vi "Initialize.vi"(8 "error in":errorcluster, 11 "Plugin in":refnum<class "MP710995.lvclass">) -> (0 "error out":errorcluster, 3 "Plugin out":refnum<class "MP710995.lvclass">)   [LabVIEW 2025, in "MP710995.lvlib" / "MP710995.lvclass"]
uses:
  MP710995.lvclass
  C:/Program Files/National Instruments/LabVIEW 2025/vi.lib/FlexLogger/SDK/PluginSDK.lvlibp/PEFClasses/SDK/Plugin/Plugin.lvclass
  <vilib>/FlexLogger/SDK/PluginSDK.lvlibp/PEFClasses/SDK/Processing Element/Timing Parameters.ctl
  <vilib>/FlexLogger/SDK/PluginSDK.lvlibp/PEFClasses/SDK/Processing Element/Timing Method.ctl
  <vilib>/FlexLogger/SDK/PluginSDK.lvlibp/PEFClasses/SDK/Channel/Data Type.ctl
  MP710995.lvclass/MP710995.ctl
  <vilib>/FlexLogger/SDK/PluginSDK.lvlibp/PEFClasses/SDK/Setpoint Consumer Channel/Setpoint Consumer Channel.lvclass
  C:/Program Files/National Instruments/LabVIEW 2025/vi.lib/FlexLogger/SDK/PluginSDK.lvlibp/PEFClasses/SDK/Channel/Channel.lvclass
  <vilib>/FlexLogger/SDK/PluginSDK.lvlibp/PEFClasses/SDK/Producer Channel/Producer Channel.lvclass
  <vilib>/FlexLogger/SDK/PluginSDK.lvlibp/PEFClasses/SDK/Plugin/ParameterAccess/Write String.vi
  <vilib>/FlexLogger/SDK/PluginSDK.lvlibp/PEFClasses/SDK/Setpoint Consumer Channel/Create Setpoint Consumer Channel.vi
  <vilib>/FlexLogger/SDK/PluginSDK.lvlibp/PEFClasses/SDK/Producer Channel/Create Producer Channel_v2.vi
  <vilib>/FlexLogger/SDK/PluginSDK.lvlibp/PEFClasses/SDK/Plugin/Plugin.lvclass
  <vilib>/FlexLogger/SDK/PluginSDK.lvlibp/PEFClasses/SDK/Channel/Channel.lvclass
  <vilib>/FlexLogger/SDK/PluginSDK.lvlibp/PEFClasses/SDK/Processing Element/Processing Element.lvclass
  <vilib>/FlexLogger/SDK/PluginSDK.lvlibp
  <vilib>/FlexLogger/SDK/PluginSDK.lvlibp/PEFClasses/SDK/Channel/ParameterAccess/Write DBL.vi
  <vilib>/FlexLogger/SDK/PluginSDK.lvlibp/PEFClasses/SDK/Channel/ParameterAccess/Write Boolean.vi
  Device Info.ctl
  C:/Program Files/National Instruments/LabVIEW 2025/vi.lib/FlexLogger/SDK/PluginSDK.lvlibp/PEFClasses/SDK/Consumer Channel/Consumer Channel.lvclass
  C:/Program Files/National Instruments/LabVIEW 2025/vi.lib/FlexLogger/SDK/PluginSDK.lvlibp/PEFClasses/SDK/Setpoint Consumer Channel/Setpoint Consumer Channel.lvclass
  C:/Program Files/National Instruments/LabVIEW 2025/vi.lib/FlexLogger/SDK/PluginSDK.lvlibp/PEFClasses/SDK/Processing Element/Processing Element.lvclass
  C:/Users/Steve/Documents/Git/MP710995-Plugin/Source/MP710995/MP710995.lvclass
panel:
  # "C:\\Program Files\\National Instruments\\LabVIEW 2025\\resource\\FlexLogger\\SDK\\PluginEnvironmentSimulator"
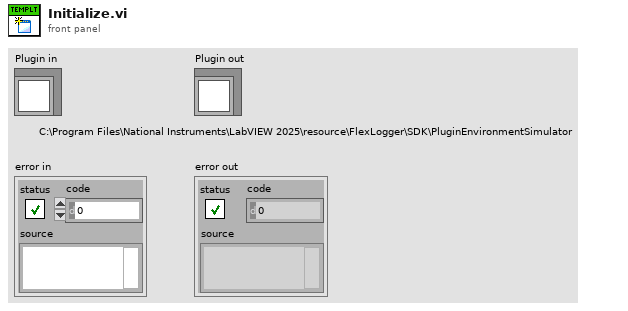
[diagram p1: front panel]
types:
  T1 = cluster{"Output":bool, "Current Limit":dbl, "Voltage":dbl, "Measured Voltage":dbl, "Measured Current":dbl, "OCP":bool}[]
  T2 = typedef "PluginSDK.lvlibp/Channel.lvclass/Data Type.ctl" = enum16{"Wfm (DBL)", "Wfm (Digital)"}
  T3 = typedef "PluginSDK.lvlibp/Processing Element.lvclass/Timing Parameters.ctl" = cluster{"Timing Method":T4, "Timing Period (ms)":i32}
  T4 = typedef "PluginSDK.lvlibp/Processing Element.lvclass/Timing Method.ctl" = enum16{"Periodic", "Immediate", "On Data Ready", "Triggered"}
  T5 = typedef "Device Info.ctl" = cluster{"Device Name":string, "Serial Number":string, "Channels":cluster{"Output":bool, "Current Limit":dbl, "Voltage":dbl, "OVP":bool, "OCP":bool}[]}
  T6 = cluster{"Output":bool, "Current Limit":dbl, "Voltage":dbl, "OVP":bool, "OCP":bool}[]
  T7 = cluster{"Output":bool, "Current Limit":dbl, "Voltage":dbl, "OVP":bool, "OCP":bool}
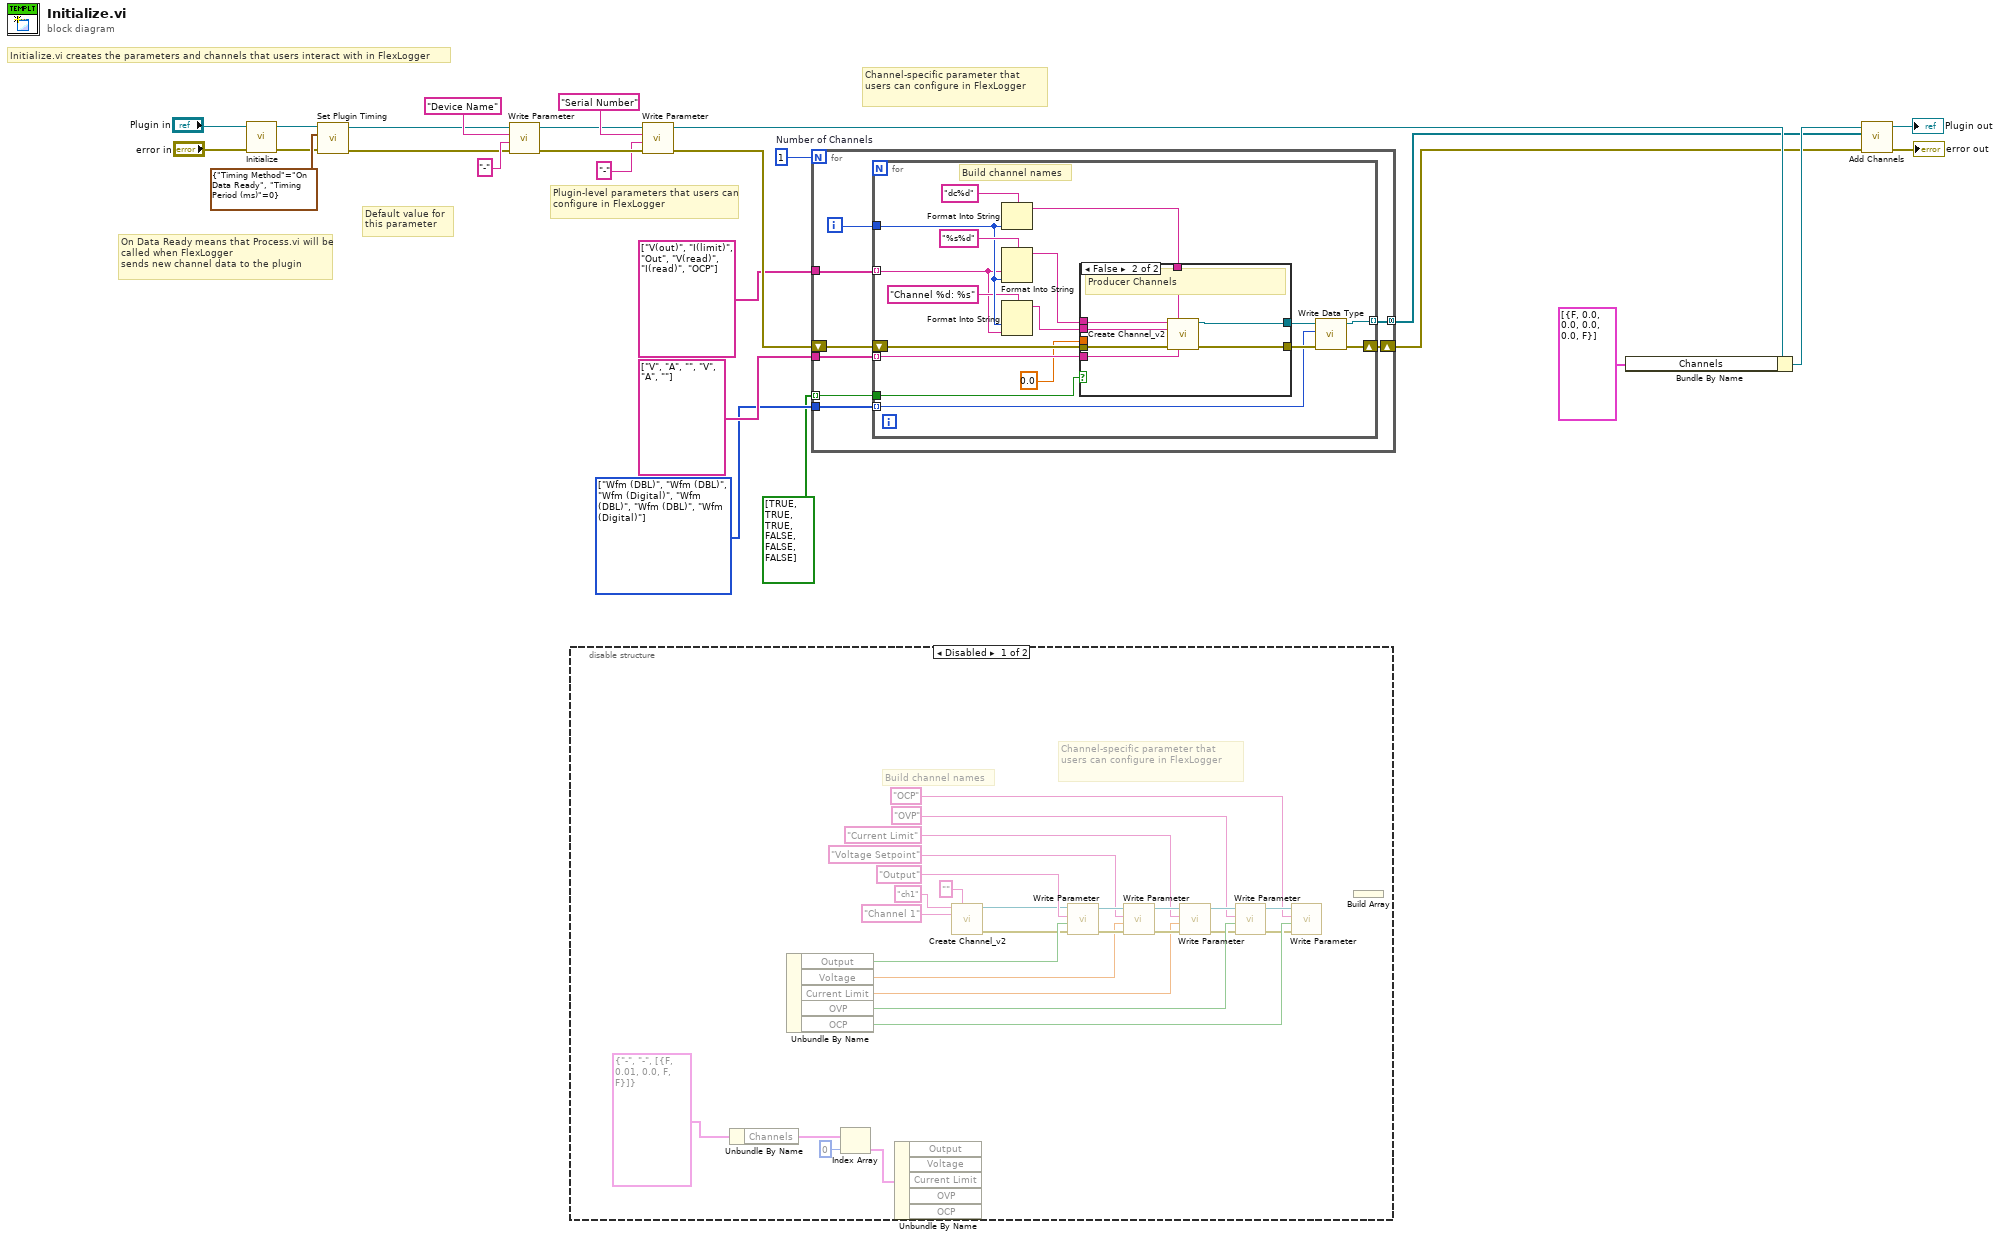
[diagram p0: block diagram]
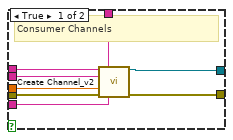
[diagram p2: hidden frame]
diagram:
  w5 = T2[] [enum."Wfm (DBL)", enum."Wfm (DBL)", enum."Wfm (Digital)", enum."Wfm (DBL)", enum."Wfm (DBL)", enum."Wfm (Digital)"] items=["Wfm (DBL)", "Wfm (Digital)"]
  w8 = 1  # Number of Channels
  # "Channel-specific parameter that users can configure in FlexLogger"
  # "Default value for this parameter"
  # "Plugin-level parameters that users can configure in FlexLogger"
  # "On Data Ready means that Process.vi will be called when FlexLogger \nsends new channel data to the plugin"
  # "Initialize.vi creates the parameters and channels that users interact with in FlexLogger"
  n1 = call-parent "Initialize.vi"("error in (no error)"="error in", "Plugin in"="Plugin in") -> ("error out"=w19:errorcluster, "Plugin out"=w18:refnum<class "MP710995.lvclass">)  [unwired: 8 in]
  n2 = call <vilib>:"Set Plugin Timing.vi"("error in (no error)"=w19, "Timing Parameters"=T3 {"Timing Method"=enum."On Data Ready", "Timing Period (ms)"=0}, "Plugin in"=w18) -> ("error out"=w11:errorcluster, "Plugin out"=w12:refnum<class "MP710995.lvclass">)  [unwired: 7 in]
  n3 = call-poly <vilib>:"Write Parameter.vi"("error in (no error)"=w11, "Value"="-", "Name"="Device Name", "Plugin in"=w12) -> ("error out"=w15:errorcluster, "Plugin out"=w16:refnum<class "MP710995.lvclass">)  [unwired: 6 in]
  n4 = disable-structure shown="Disabled" {
    frame Disabled {
      # "Channel-specific parameter that users can configure in FlexLogger"
      # "Build channel names"
      n5 = Unbundle By Name(T5 {"Device Name"="-", "Serial Number"="-", "Channels"=[{"Output"=FALSE, "Current Limit"=0.01, "Voltage"=0.0, "OVP"=FALSE, "OCP"=FALSE}]}) -> ("Channels"=w30:T6)
      n6 = Unbundle By Name() -> ("Output"=w43:bool, "Voltage"=w49:dbl, "Current Limit"=w47:dbl, "OVP"=w44:bool, "OCP"=w45:bool)  [unwired: 1 in]
      n7 = Index Array(array=w30, index=0) -> (element=w29:T7)
      n8 = Unbundle By Name(w29) -> ()  [unwired: 5 out]
      n9 = call-poly <vilib>:"Create Channel_v2.vi"("Unique Channel Identifier"="ch1" ("format string"), "Display Group"="", "Default Channel Name"="Channel 1" ("format string")) -> ("Setpoint Consumer Channel"=w35:refnum<class "Setpoint Consumer Channel.lvclass">, "error in (no error)"=w33:errorcluster, "error out"=w34:errorcluster)  [unwired: 10 in]
      n10 = call-poly <vilib>:"Write Parameter.vi"("error in (no error)"=w34, "Value"=w43, "Name"="Output", "Channel in"=w35) -> ("error out"=w50:errorcluster, "Channel out"=w51:refnum<class "Setpoint Consumer Channel.lvclass">)  [unwired: 6 in]
      n11 = call-poly <vilib>:"Write Parameter.vi"("error in (no error)"=w50, "Value"=w49, "Name"="Voltage Setpoint", "Channel in"=w51) -> ("error out"=w53:errorcluster, "Channel out"=w52:refnum<class "Setpoint Consumer Channel.lvclass">)  [unwired: 6 in]
      n12 = call-poly <vilib>:"Write Parameter.vi"("error in (no error)"=w53, "Value"=w47, "Name"="Current Limit", "Channel in"=w52) -> ("error out"=w39:errorcluster, "Channel out"=w38:refnum<class "Setpoint Consumer Channel.lvclass">)  [unwired: 6 in]
      n13 = call-poly <vilib>:"Write Parameter.vi"("error in (no error)"=w39, "Value"=w44, "Name"="OVP", "Channel in"=w38) -> ("error out"=w41:errorcluster, "Channel out"=w40:refnum<class "Setpoint Consumer Channel.lvclass">)  [unwired: 6 in]
      n14 = call-poly <vilib>:"Write Parameter.vi"("error in (no error)"=w41, "Value"=w45, "Name"="OCP", "Channel in"=w40) -> ()  [unwired: 6 in, 2 out]
      n15 = Build Array() -> ()  [unwired: 1 in, 1 out]
    }
    frame Enabled {
    }
  }
  n16 = call-poly <vilib>:"Write Parameter.vi"("error in (no error)"=w15, "Value"="-", "Name"="Serial Number", "Plugin in"=w16) -> ("error out"=w13:errorcluster, "Plugin out"=w10:refnum<class "MP710995.lvclass">)  [unwired: 6 in]
  n17 = for {
    N: w8 -> [_]
    tunnel: string[] ["V(out)", "I(limit)", "Out", "V(read)", "I(read)", "OCP"] -> [w60]
    tunnel: string[] ["V", "A", "", "V", "A", ""] -> [w59]
    tunnel: w5 -> [w58]
    shift-right: [w57] -> w3
    shift-left: w13 -> [w62]
    tunnel: [w56] -> w4 mode=concatenating
    tunnel: bool[] [TRUE, TRUE, TRUE, FALSE, FALSE, FALSE] -> [w55] mode=indexing
    i -> [w61]
    n18 = for {
      tunnel: w61 -> [w74]
      tunnel: w60 -> [w72] mode=indexing
      tunnel: w59 -> [w70] mode=indexing
      tunnel: w58 -> [w66] mode=indexing
      shift-right: [w67] -> w57
      shift-left: w62 -> [w79]
      tunnel: [w65] -> w56 mode=indexing
      tunnel: w55 -> [w63]
      # "Build channel names"
      n19 = Format Into String(format string="dc%d", w74) -> (resulting string=w76:string)  [unwired: 2 in, 1 out]
      n20 = Format Into String(format string="%s%d", w72, w74) -> (resulting string=w77:string)  [unwired: 2 in, 1 out]
      n21 = Format Into String(format string="Channel %d: %s", w74, w72) -> (resulting string=w71:string)  [unwired: 2 in, 1 out]
      n22 = case shown="False" w63 {
        tunnel: w79 -> [w87 w94]
        tunnel: w77 -> [w86 w93]
        tunnel: w76 -> [w85 w92]
        tunnel: w71 -> [w84 w91]
        tunnel: w70 -> [w83 w90]
        tunnel: 0.0 ("Default Value") -> [w82 _]
        tunnel: [w81 w89] -> w68
        tunnel: [w80 w88] -> w64
        frame True {
          # "Consumer Channels"
          n23 = call-poly <vilib>:"Create Channel_v2.vi"("Unique Channel Identifier"=w86, "Display Group"=w85, "Default Channel Name"=w84, "Default Value"=w82, "error in (no error)"=w87, "Unit"=w83) -> ("Setpoint Consumer Channel"=w80:refnum<class "Setpoint Consumer Channel.lvclass">, "error out"=w81:errorcluster)  [unwired: 8 in]
        }
        frame False {
          # "Producer Channels"
          n24 = call-poly <vilib>:"Create Channel_v2.vi"("Unique Channel Identifier"=w93, "Display Group"=w92, "Default Channel Name"=w91, "error in (no error)"=w94, "Unit"=w90) -> ("Producer Channel"=w88:refnum<class "Producer Channel.lvclass">, "error out"=w89:errorcluster)  [unwired: 9 in]
        }
      }
      n25 = call-dynamic "Write Data Type.vi"("error in (no error)"=w68, "Data Type"=w66, "Channel in"=w64) -> ("error out"=w67:errorcluster, "Channel out"=w65:refnum<class "Channel.lvclass">)  [unwired: 7 in]
    }
  }
  n26 = Bundle By Name(cluster=w10, "Channels"=T1 [{"Output"=FALSE, "Current Limit"=0.0, "Voltage"=0.0, "Measured Voltage"=0.0, "Measured Current"=0.0, "OCP"=FALSE}] ("Device Information.Channels")) -> (w9:refnum<class "MP710995.lvclass">)
  n27 = call <vilib>:"Add Channels.vi"("error in (no error)"=w3, "Channels"=w4, "Plugin in"=w9) -> ("error out"=→"error out":errorcluster, "Plugin out"=→"Plugin out":refnum<class "MP710995.lvclass">)  [unwired: 7 in]
